vi "Write Connection Status 2.vi"(10 "Connection Status":bool, 11 "CCD in":refnum<class "CCD.lvclass">) -> (3 "CCD out":refnum<class "CCD.lvclass">)   [LabVIEW 2016, in "Hardware.lvlib" / "CCD.lvlib" / "CCD.lvclass"]
uses:
  <userlib>/Common Components/Hardware/CCD/CCD/CCD.lvclass
  <userlib>/Common Components/Hardware/CCD/CCD/CCD.lvclass/CCD.ctl
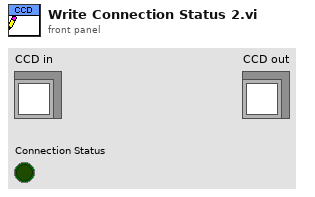
[diagram p1: front panel]
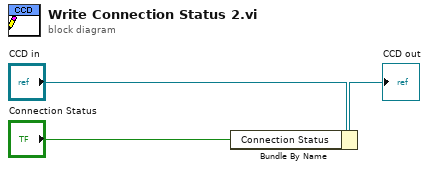
[diagram p0: block diagram]
diagram:
  n1 = Bundle By Name(cluster="CCD in", "Connection Status"="Connection Status") -> (→"CCD out":refnum<class "CCD.lvclass">)
